vi "DestroyPublicEvents.vi"(8 "error in (no error)":errorcluster, 11 "Subsystem":refnum<class "DAQmx(AI).lvclass">) -> (0 "error out":errorcluster, 3 "Subsystem out":refnum<class "DAQmx(AI).lvclass">)   [LabVIEW 2013, in "DAQmx(AI).lvclass"]
doc: "JKI State Machine Objects (SMO) 1.0.0.5\nJKI - JKI\nCopyright (c) 2016, JKI"
uses:
  DAQmx(AI).lvclass
  <vilib>/JKI/JKI SMO/SMO/SMO.lvclass
panel:
  # "For instructions on how to use the JKI State Machine Objects, examples and video tutorials, visit:\nhttp://jki.net/state-machine-objects/\n\nJKI State Machine Objects™\nhttp://jki.net/state-machine-objects/\nCopyright (C) 2005-2015, JKI <info@jki.net>\nALL RIGHTS RESERVED"
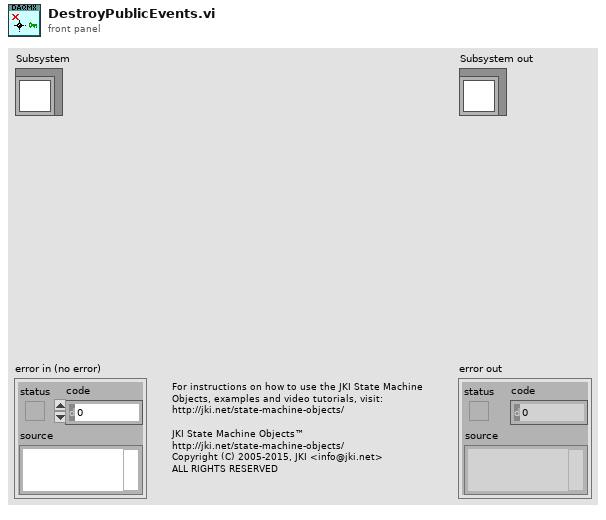
[diagram p1: front panel]
types:
  T1 = typedef "DAQmx(AI).lvclass/PublicEvents--Cluster.ctl" = cluster{"Value Changed":refnum<user-event>, "Task Configuration":refnum<user-event>, "Scaling":refnum<user-event>}
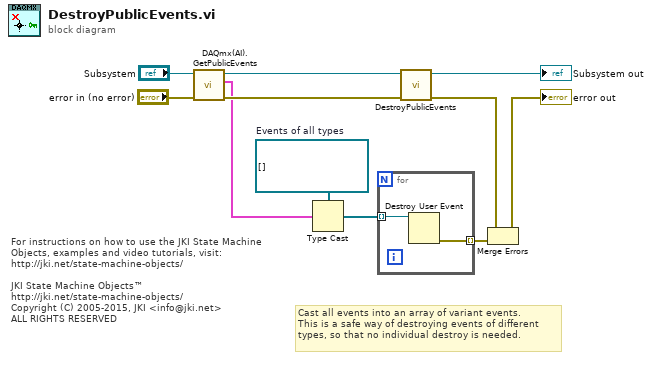
[diagram p0: block diagram]
diagram:
  w3 = refnum<user-event>[] []  # Events of all types
  # "For instructions on how to use the JKI State Machine Objects, examples and video tutorials, visit:\nhttp://jki.net/state-machine-objects/\n\nJKI State Machine Objects™\nhttp://jki.net/state-machine-objects/\nCopyright (C) 2005-2015, JKI <info@jki.net>\nALL RIGHTS RESERVED"
  # "Cast all events into an array of variant events.\nThis is a safe way of destroying events of different\ntypes, so that no individual destroy is needed."
  n1 = call "DAQmx(AI).GetPublicEvents.vi"("error in (no error)"="error in (no error)", "Subsystem"="Subsystem") -> ("error out"=w7:errorcluster, "DAQmx(AI) Public Events"=w1:T1, "Subsystem out"=w9:refnum<class "DAQmx(AI).lvclass">)  [unwired: 7 in]
  n2 = Type Cast(type=w3, x=w1) -> (*(type *) &x=w4:refnum<user-event>[])
  n3 = for {
    tunnel: w4 -> [w13] mode=indexing
    tunnel: [w12] -> w2 mode=indexing
    n4 = Destroy User Event(user event=w13) -> (error out=w12:errorcluster)  [unwired: 1 in]
  }
  n5 = call-parent "DestroyPublicEvents.vi"("error in (no error)"=w7, "SMO"=w9) -> ("error out"=w6:errorcluster, "SMO out"=→"Subsystem out":refnum<class "DAQmx(AI).lvclass">)  [unwired: 8 in]
  n6 = Merge Errors(w6, w2) -> (→"error out":errorcluster)
